vi "Hatch & Cargo Control.vi"() -> ()   [LabVIEW 2018]
uses:
  <vilib>/Rock Robotics/WPI/ThirdParty/Phoenix-LabVIEW/Motor Controller/Controls/CTRE_Phoenix_MotorControl_NeutralMode.ctl
  <vilib>/Rock Robotics/WPI/ThirdParty/Phoenix-LabVIEW/Motor Controller/Controls/CTRE_Phoenix_MotorControl_ControlMode.ctl
  Infrastructure/RobotMap.vi
  Infrastructure/Constants.vi
  <vilib>/Rock Robotics/Network Tables/NT Read Boolean.vi
  Robot Global Data.vi
  <vilib>/Rock Robotics/WPI/ThirdParty/Phoenix-LabVIEW/Motor Controller/Get/CTRE_Phoenix_MotorController_GetSelectedSensorData.vi
  <vilib>/Rock Robotics/Network Tables/NT Write Number.vi
  <vilib>/Rock Robotics/WPI/ThirdParty/Phoenix-LabVIEW/Motor Controller/Get/CTRE_Phoenix_MotorController_GetOutputCurrent_Enhanced.vi
panel:
  in  "Cargo Current Threshold when the ball is in intake":dbl=5.0
  out "Hatch Velocity":i32(graph)
  out "Hatch Position":i32(graph)
  # "Not an actual number atm"
  # "Cargo Positive Must Be IN"
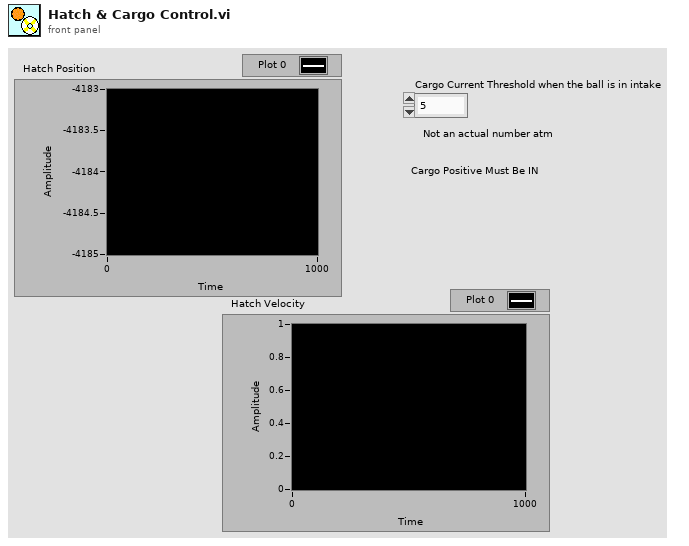
[diagram p1: front panel]
types:
  T1 = typedef "CTRE_Phoenix_MotorControl_NeutralMode.ctl" = enum8{"EEPROMSetting", "Override to Coast", "Override to Brake"}
  T2 = typedef "WPI_MotorControlDeviceRef.ctl" = cluster{"DeviceStatus":errorcluster, "Type":T3, "PWM":cluster{"PWM Channel":T4, "DeadBand":T5}, "CAN":cluster{"Device Number":u8, "SetOutput VI Ref":variant, "GetOutput VI Ref":variant, "Enable VI Ref":variant, "Disable VI Ref":variant, "Data":variant}, "Invert":bool, "DIO PWM":cluster{"PWM \"Enable\" Channel":T4, "DIOChannel":T6, "PWM Rate":dbl}}
  T3 = typedef "WPI_MotorControlType.ctl" = enum16{"PWM", "CAN", "DIO PWM"}
  T4 = typedef "FPGA_DIOPWMChannel.ctl" = enum8{"PWM 0", "PWM 1", "PWM 2", "PWM 3", "PWM 4", "PWM 5", "PWM 6", "PWM 7", "PWM 8", "PWM 9", "PWM MXP 0", "PWM MXP 1", "PWM MXP 2", "PWM MXP 3", "PWM MXP 4", "PWM MXP 5", "PWM MXP 6", "PWM MXP 7", "PWM MXP 8", "PWM MXP 9", "Invalid"}
  T5 = typedef "WPI_PWMDeadband.ctl" = cluster{"Name":string, "maxPositivePwm":i32, "minPositivePwm":i32, "centerPwm":i32, "maxNegativePwm":i32, "minNegativePwm":i32, "angularRange":u16}
  T6 = typedef "FPGA_DIOChannel.ctl" = enum8{"DIO 0", "DIO 1", "DIO 2", "DIO 3", "DIO 4", "DIO 5", "DIO 6", "DIO 7", "DIO 8", "DIO 9", "DIO MXP 0", "DIO MXP 1", "DIO MXP 2", "DIO MXP 3", "DIO MXP 4", "DIO MXP 5", "DIO MXP 6", "DIO MXP 7", "DIO MXP 8", "DIO MXP 9", "DIO MXP 10", "DIO MXP 11", "DIO MXP 12", "DIO MXP 13", "DIO MXP 14", "DIO MXP 15", "SPI Port CS1", "SPI Port CS2", "SPI Port CS3", "SPI Port MISO", "SPI Port MOSI", "Invalid"}
  T7 = cluster{"P":dbl, "I":dbl, "D":dbl, "F":dbl, "I Zone":dbl}
  T8 = typedef "CTRE_Phoenix_MotorControl_ControlMode.ctl" = u16
  T9 = cluster{"Cargo Motor Value":dbl, "Hatch Setpoint":dbl}
  T10 = cluster{"Position (Raw Sensor Units)":i32, "Velocity (Raw Sensor Units per 100 ms)":i32}
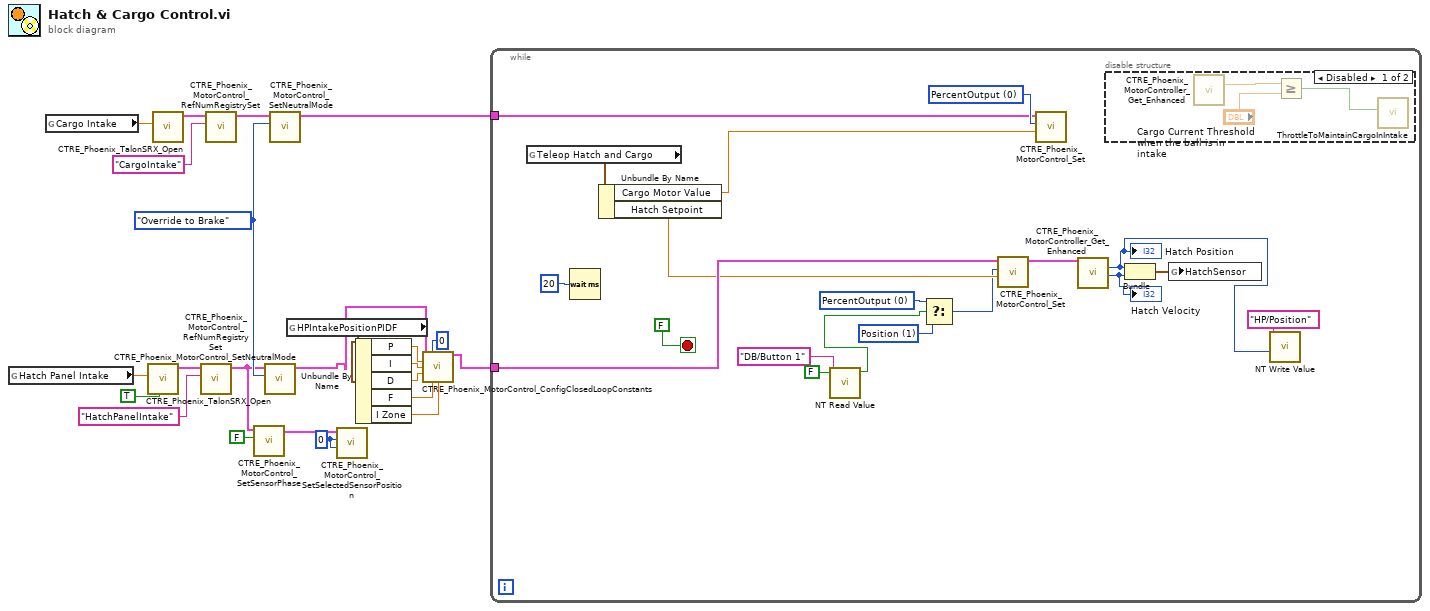
[diagram p0: block diagram]
diagram:
  w2 = 0 ("New Sensor Position")
  w16 = CTRE_Phoenix_MotorControl_NeutralMode."Override to Brake" ("Motor Control Neutral Mode")
  n1 = global read "RobotMap.vi" "Hatch Panel Intake"() -> (w20:dbl)
  n2 = global read "RobotMap.vi" "Cargo Intake"() -> (w21:dbl)
  n3 = call <vilib>:"CTRE_Phoenix_TalonSRX_Open.vi"("Invert"=TRUE, "Device Number"=w20) -> ("CAN Talon SRX Ref"=w22:T2)  [unwired: 8 in, 1 out]
  n4 = call <vilib>:"CTRE_Phoenix_TalonSRX_Open.vi"("Device Number"=w21) -> ("CAN Talon SRX Ref"=w23:T2)  [unwired: 9 in, 1 out]
  n5 = call <vilib>:"CTRE_Phoenix_MotorControl_RefNumRegistrySet.vi"("refnum name"="HatchPanelIntake", "PhoenixMotorControlDevRef"=w22) -> ("PhoenixMotorControlDevRef"=w5:T2)  [unwired: 8 in, 1 out]
  n6 = call <vilib>:"CTRE_Phoenix_MotorControl_RefNumRegistrySet.vi"("refnum name"="CargoIntake", "PhoenixMotorControlDevRef"=w23) -> ("PhoenixMotorControlDevRef"=w17:T2)  [unwired: 8 in, 1 out]
  n7 = call <vilib>:"CTRE_Phoenix_MotorControl_SetSensorPhase.vi"("PhaseSensor"=FALSE, "PhoenixMotorControlDevRef"=w5) -> ("PhoenixMotorControlDevRef"=w3:T2)  [unwired: 8 in, 1 out]
  n8 = call <vilib>:"CTRE_Phoenix_MotorControl_SetNeutralMode.vi"("Motor Control Neutral Mode"=w16, "PhoenixMotorControlDevRef"=w5) -> ("PhoenixMotorControlDevRef"=w6:T2)  [unwired: 8 in, 1 out]
  n9 = call <vilib>:"CTRE_Phoenix_MotorControl_SetNeutralMode.vi"("Motor Control Neutral Mode"=w16, "PhoenixMotorControlDevRef"=w17) -> ("PhoenixMotorControlDevRef"=w14:T2)  [unwired: 8 in, 1 out]
  n10 = global read "Constants.vi" "HPIntakePositionPIDF"() -> (w13:T7)
  n11 = call <vilib>:"CTRE_Phoenix_MotorControl_SetSelectedSensorPosition.vi"("pidLoopIdx"=w2, "New Sensor Position"=w2, "PhoenixMotorControlDevRef"=w3) -> ()  [unwired: 7 in, 2 out]
  n12 = Unbundle By Name(w13) -> ("P"=w12:dbl, "I"=w11:dbl, "D"=w10:dbl, "F"=w9:dbl, "I Zone"=w8:dbl)
  n13 = call <vilib>:"CTRE_Phoenix_MotorControl_ConfigClosedLoopConstants.vi"("PhoenixMotorControlDevRef"=w6, "slotIdx"=0, "P"=w12, "I"=w11, "D"=w10, "F"=w9, "I Zone"=w8) -> ("PhoenixMotorControlDevRef"=w15:T2)  [unwired: 7 in, 1 out]
  n14 = while {
    tunnel: w15 -> [w39]
    tunnel: w14 -> [w35]
    stop <- FALSE stop-if-true
    w28 = T8 1 items=["PercentOutput"=0, "Position"=1, "Velocity"=2, "Current"=3, "Follower"=5, "MotionProfile"=6, "MotionMagic"=7, "MotionProfileArc"=10, "Disabled"=15] ("Control Mode")
    w29 = T8 0 items=["PercentOutput"=0, "Position"=1, "Velocity"=2, "Current"=3, "Follower"=5, "MotionProfile"=6, "MotionMagic"=7, "MotionProfileArc"=10, "Disabled"=15] ("Control Mode")
    w42 = T8 0 items=["PercentOutput"=0, "Position"=1, "Velocity"=2, "Current"=3, "Follower"=5, "MotionProfile"=6, "MotionMagic"=7, "MotionProfileArc"=10, "Disabled"=15] ("Control Mode")
    n15 = global read "Robot Global Data.vi" "Teleop Hatch and Cargo"() -> (w38:T9)
    n16 = Wait (ms)(milliseconds to wait=u32 20) -> ()  [unwired: 1 out]
    n17 = Unbundle By Name(w38) -> ("Cargo Motor Value"=w36:dbl, "Hatch Setpoint"=w37:dbl)
    n18 = call-poly <vilib>:"NT Read Value.vi"("Default Value"=FALSE, "Name"="DB/Button 1") -> ("Boolean"=w27:bool)  [unwired: 8 in, 1 out]
    n19 = Select(t=w29, s=w27, f=w28) -> (s? t:f=w30:T8)
    n20 = call <vilib>:"CTRE_Phoenix_MotorControl_Set.vi"("Output"=w37, "Control Mode"=w30, "PhoenixMotorControlDevRef"=w39) -> ("PhoenixMotorControlDevRef"=w34:T2)  [unwired: 7 in, 1 out]
    n21 = call <vilib>:"CTRE_Phoenix_MotorControl_Set.vi"("Output"=w36, "Control Mode"=w42, "PhoenixMotorControlDevRef"=w35) -> ()  [unwired: 7 in, 2 out]
    n22 = call-poly <vilib>:"CTRE_Phoenix_MotorController_Get_Enhanced.vi"("PhoenixMotorControlDevRef"=w34) -> ("Position (Raw Sensor Units)"=w24:i32, "Velocity (Raw Sensor Units per 100 ms)"=w32:i32)  [unwired: 11 in, 2 out]
    "Hatch Position" <- w24
    "Hatch Velocity" <- w32
    n23 = disable-structure shown="Disabled" {
      frame Disabled {
        n24 = call-poly <vilib>:"CTRE_Phoenix_MotorController_Get_Enhanced.vi"() -> ("Output Current"=w45:dbl)  [unwired: 13 in, 2 out]
        n25 = Greater Or Equal?(x=w45, y="Cargo Current Threshold when the ball is in intake") -> (x >= y?=w43:bool)
        n26 = call "ThrottleToMaintainCargoInIntake.vi"("Current above threshold?"=w43) -> ()  [unwired: 10 in, 1 out]
      }
      frame Enabled {
      }
    }
    n27 = Bundle("Position (Raw Sensor Units)"=w24, "Velocity (Raw Sensor Units per 100 ms)"=w32) -> (w33:T10)  [unwired: 1 in]
    n28 = global write "Robot Global Data.vi" "HatchSensor"(w33) -> ()
    n29 = call-poly <vilib>:"NT Write Value.vi"("Numeric"=w24, "Name"="HP/Position") -> ()  [unwired: 9 in, 1 out]
  }
